vi "系统设置_古田户外.vi"() -> ()   [LabVIEW 2016]
uses:
  <vilib>/Utility/miscctls.llb/LVPointTypeDef.ctl
  <vilib>/Utility/config.llb/Read Key (U32).vi
  <vilib>/Utility/config.llb/Write Key (I32).vi
  PLC/PLC.lvlib
  <vilib>/ptbypt/NI_PtbyPt.lvlib
  <vilib>/Utility/config.llb/NI_LVConfig.lvlib
panel:
  in  "运行模式":enum16{"维护模式", "常规模式", "应急模式", "质控模式"}(ring)
  in  "运行间隔":i16=4 min=1 max=24
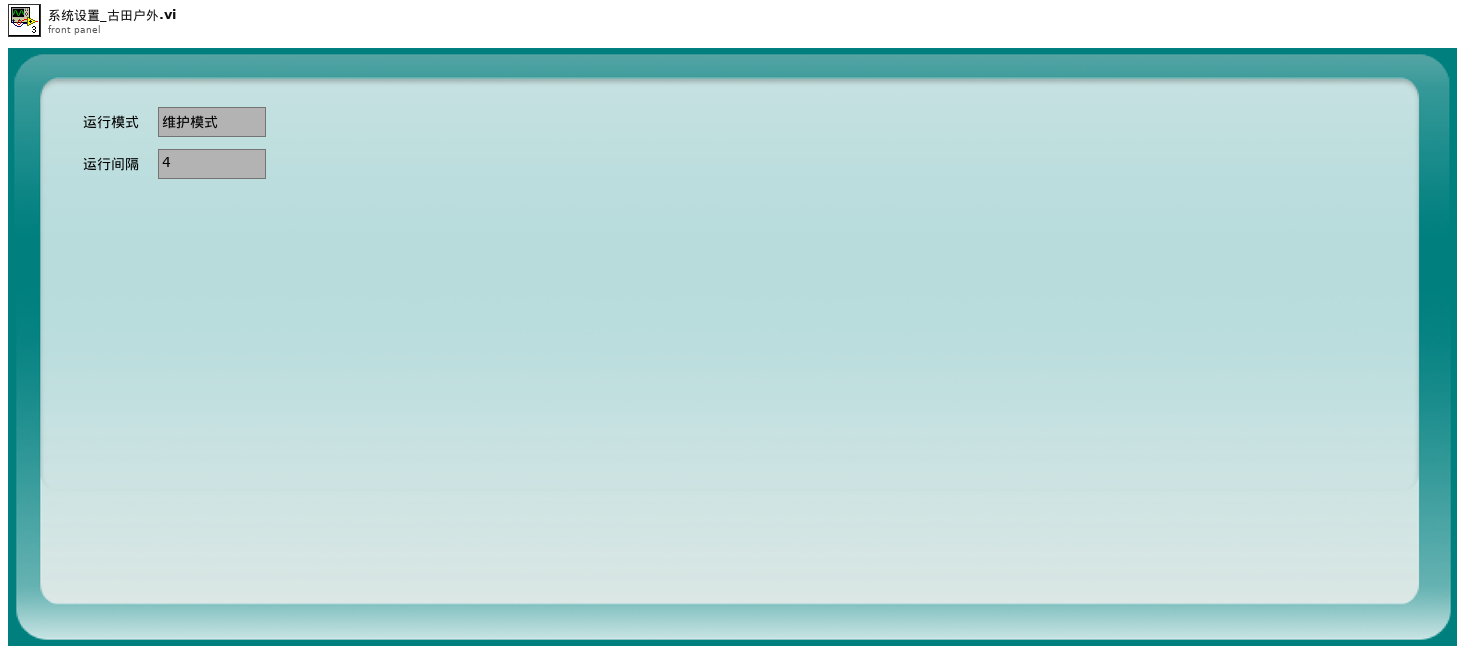
[diagram p1: front panel]
types:
  T1 = typedef "LVPointTypeDef.ctl" = cluster{"Horizontal":i16, "Vertical":i16}
  T2 = typedef "NI_LVConfig.lvlib/Config Data RefNum.ctl" = refnum<k1>
  T3 = enum16{"水样测量", "标样核查", "零点核查", "加标回收", "平行样", "校零", "校标"}
  T4 = cluster{"是否启用仪器":bool, "CODMn":cluster{"启动测量模式":cluster{"测量模式":enum16{"水样测量", "标样核查", "零点核查", "加标回收", "平行样", "校零", "校标"}}, "确定按钮":bool}}
  T5 = typedef "LVDateTimeRec.ctl" = cluster{"秒数的小数部分":dbl, "秒":i32, "分":i32, "时":i32, "日":i32, "月":i32, "年":i32, "天数（周）":i32, "天数（年）":i32, "DST":i32}
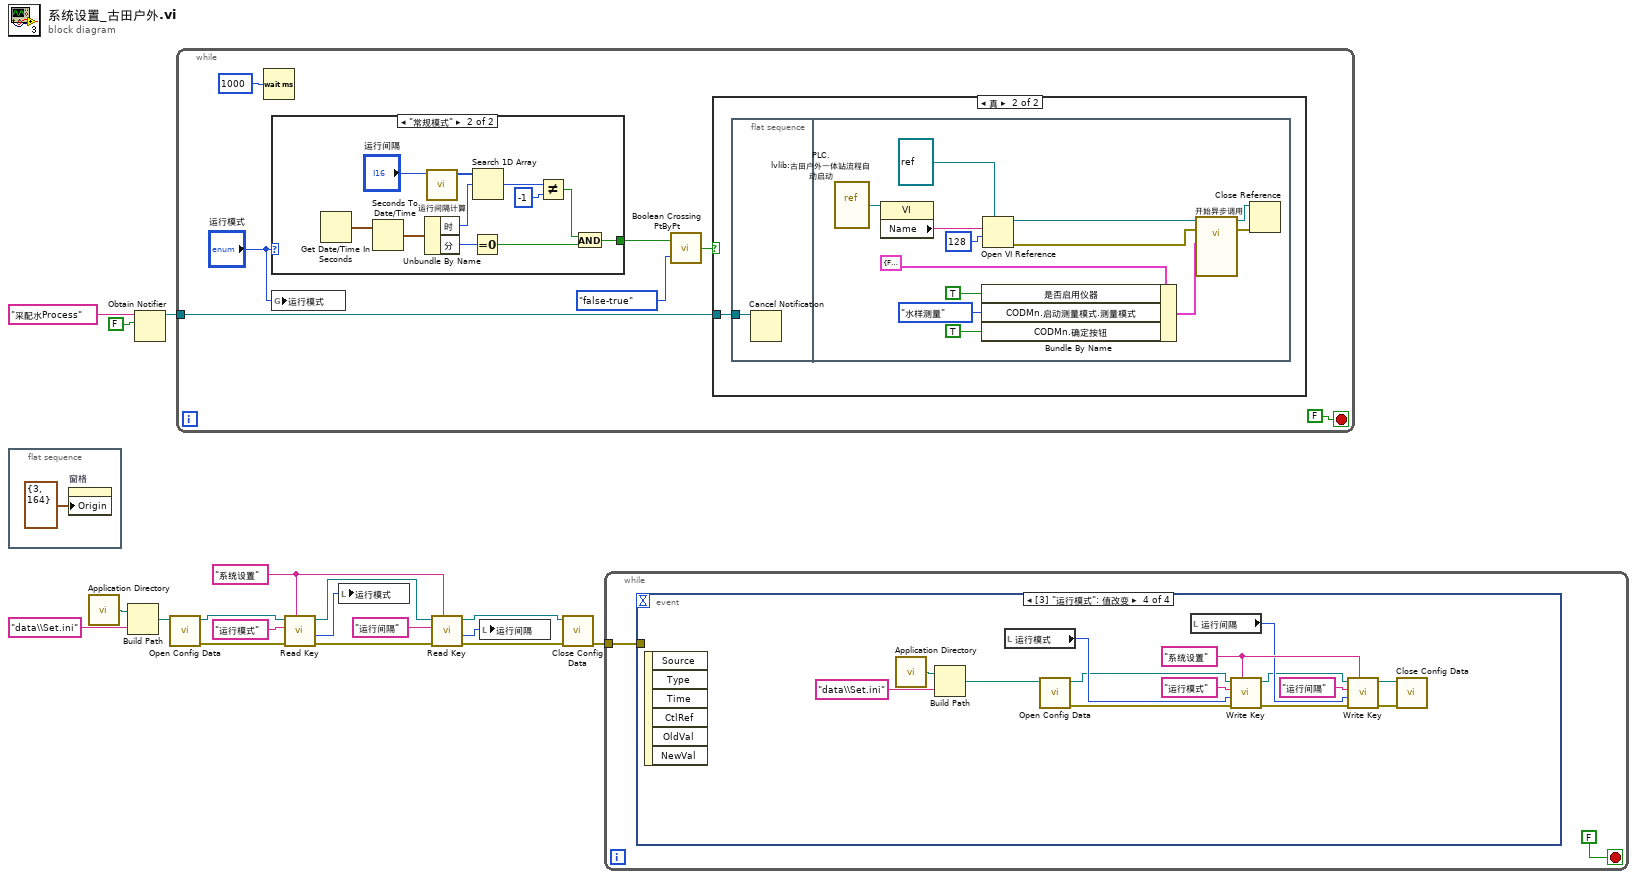
[diagram p0: block diagram]
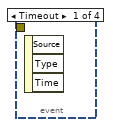
[diagram p4: hidden frame]
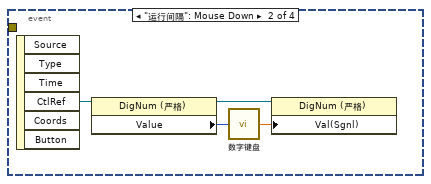
[diagram p5: hidden frame]
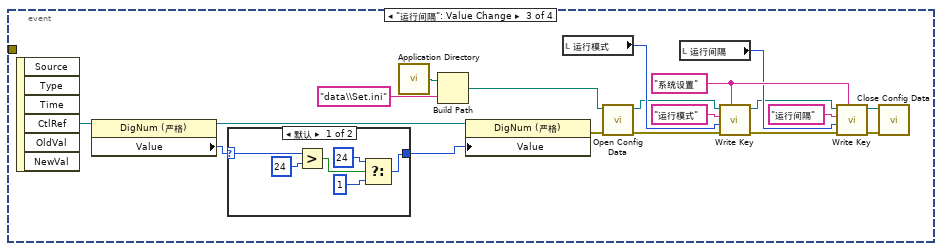
[diagram p6: hidden frame]
diagram:
  w1 = "系统设置" ("section")
  n1 = flat-sequence {
    frame #0 {
      n2 = property on="窗格" class="Pane"("Origin"=T1 {"Horizontal"=3, "Vertical"=164} ("原点")) -> ()  [unwired: 2 in, 2 out]
    }
  }
  n3 = call <vilib>:"Application Directory.vi"() -> ("Application Directory"=w13:path)
  n4 = Build Path(base path=w13, name or relative path="data\\Set.ini" ("名称或相对路径")) -> (appended path=w11:path)
  n5 = Obtain Notifier(name (unnamed)="采配水Process" ("名称（未命名）"), notification data type=FALSE) -> (notifier out=w16:refnum<notifier>)  [unwired: 2 in, 2 out]
  n6 = call <vilib>:"Open Config Data.vi"("configuration file path"=w11) -> ("error out"=w14:errorcluster, "refnum"=w15:T2)  [unwired: 8 in, 1 out]
  n7 = while {
    tunnel: w16 -> [w24]
    stop <- FALSE stop-if-true
    n8 = Wait (ms)(milliseconds to wait=u32 1000 ("等待时间（毫秒）")) -> ()  [unwired: 1 out]
    n9 = case shown="\"常规模式\"" "运行模式" {
      tunnel: [_ w42] -> w23
      frame "维护模式", Default {
      }
      frame "常规模式" {
        n10 = Get Date/Time In Seconds() -> (seconds since 1Jan1904=w51:timestamp)
        n11 = Seconds To Date/Time(time stamp (now)=w51) -> (date time rec=w50:T5)  [unwired: 1 in]
        n12 = Unbundle By Name(w50) -> ("时"=w47:i32, "分"=w49:i32)
        n13 = call "运行间隔计算.vi"("运行周期"="运行间隔") -> ("数组"=w48:i32[])  [unwired: 10 in]
        n14 = Equal To 0?(x=w49) -> (x = 0?=w43:bool)
        n15 = Search 1D Array(1D array=w48, element=w47) -> (index of element=w46:i32)  [unwired: 1 in]
        n16 = Not Equal?(x=w46, y=-1) -> (x != y?=w44:bool)
        n17 = And(x=w44, y=w43) -> (x .and. y?=w42:bool)
      }
    }
    n18 = global write "系统变量.vi" "运行模式"("运行模式") -> ()
    n19 = call <vilib>:"Boolean Crossing PtByPt.vi"("direction"=enum16{"either", "false-true", "true-false"}."false-true", "input"=w23) -> ("crossing"=w21:bool)  [unwired: 1 in]
    n20 = case shown="真" w21 {
      tunnel: w24 -> [_ w27]
      frame False {
      }
      frame True {
        n21 = flat-sequence {
          tunnel: w27 -> [w28]
          frame #0 {
            n22 = Cancel Notification(0:w28) -> ()  [unwired: 1 in, 3 out]
          }
          frame #1 {
            n23 = vi-ref "PLC.lvlib:古田户外一体站流程自动启动.vi"() -> (w41:refnum<vi>)
            n24 = property class="VI"(reference=w41) -> ("Name"=w40:string)  [unwired: 1 in, 2 out]
            n25 = Bundle By Name(cluster=T4 {"是否启用仪器"=FALSE, "CODMn"={"启动测量模式"={"测量模式"=enum."水样测量"}, "确定按钮"=FALSE}} ("参数"), "是否启用仪器"=TRUE, "CODMn.启动测量模式.测量模式"=T3."水样测量", "CODMn.确定按钮"=TRUE) -> (w30:T4)
            n26 = Open VI Reference(type specifier VI Refnum (for type only)=refnum<vi> refnum, vi path=w40, options=128 ("选项")) -> (vi reference=w38:refnum<vi>, error out=w35:errorcluster)  [unwired: 3 in]
            n27 = call-by-ref "开始异步调用"(reference=w38, error in=w35, "参数"=w30) -> (reference out=w36:refnum<vi>, error out=w34:errorcluster)  [unwired: 11 in]
            n28 = Close Reference(reference=w36, error in (no error)=w34) -> ()  [unwired: 1 out]
          }
        }
      }
    }
  }
  n29 = call-poly <vilib>:"Read Key.vi"("section"=w1, "error in (no error)"=w14, "key"="运行模式" ("section"), "refnum"=w15) -> ("error out"=w7:errorcluster, "value"=w10:u32, "refnum out"=w9:T2)  [unwired: 4 in, 1 out]
  n30 = local write "运行模式"(w10) -> ()
  n31 = call-poly <vilib>:"Read Key.vi"("section"=w1, "error in (no error)"=w7, "key"="运行间隔" ("section"), "refnum"=w9) -> ("error out"=w6:errorcluster, "value"=w3:u32, "refnum out"=w8:T2)  [unwired: 4 in, 1 out]
  n32 = local write "运行间隔"(w3) -> ()
  n33 = call <vilib>:"Close Config Data.vi"("error in (no error)"=w6, "refnum"=w8) -> ("error out"=w2:errorcluster)  [unwired: 8 in, 1 out]
  n34 = while {
    tunnel: w2 -> [w53]
    stop <- FALSE stop-if-true
    n35 = event shown="[3] \"运行模式\": 值改变" {
      selector: _ -> [_ _ _ _]
      dyn-events: _ -> [_ _ _ _]
      timeout: _ -> [_ _ _ _]
      tunnel: w53 -> [_ _ _ _]
      event Timeout {
        n36 = event-data() -> ()  [unwired: 1 in, 3 out]
      }
      event "运行间隔": Mouse Down {
        n37 = event-data() -> ("CtlRef"=w55:refnum<vi>)  [unwired: 1 in, 5 out]
        n38 = property class="DigNum (严格)"(reference=w55) -> (reference out=w57:refnum<vi>, "Value"=w56:i16)  [unwired: 1 in, 1 out]
        n39 = call "数字键盘.vi"("OldNumber"=w56) -> ("NewNumber"=w58:sgl)
        n40 = property class="DigNum (严格)"(reference=w57, "Val(Sgnl)"=w58) -> ()  [unwired: 1 in, 2 out]
      }
      event "运行间隔": Value Change {
        w73 = "系统设置" ("section")
        n41 = event-data() -> ("CtlRef"=w77:refnum<vi>)  [unwired: 1 in, 5 out]
        n42 = property class="DigNum (严格)"(reference=w77) -> (reference out=w75:refnum<vi>, "Value"=w76:i16)  [unwired: 1 in, 1 out]
        n43 = case shown="默认" w76 {
          selector: w76 -> [w80 w84]
          tunnel: [w79 w84] -> w74
          frame Default {
            n44 = Greater?(x=w80, y=i16 24) -> (0:w82:bool)
            n45 = Select(t=i16 24 ("y"), s=w82, f=i16 1) -> (s? t:f=w79:i16)
          }
          frame 1..24 {
          }
        }
        n46 = call <vilib>:"Application Directory.vi"() -> ("Application Directory"=w68:path)
        n47 = Build Path(base path=w68, name or relative path="data\\Set.ini" ("名称或相对路径")) -> (appended path=w66:path)
        n48 = property class="DigNum (严格)"(reference=w75, "Value"=w74) -> (error out=w59:errorcluster)  [unwired: 1 in, 1 out]
        n49 = local read "运行模式"() -> (w71:enum16{"维护模式", "常规模式", "应急模式", "质控模式"})
        n50 = call <vilib>:"Open Config Data.vi"("error in (no error)"=w59, "configuration file path"=w66) -> ("error out"=w69:errorcluster, "refnum"=w70:T2)  [unwired: 7 in, 1 out]
        n51 = local read "运行间隔"() -> (w72:i16)
        n52 = call-poly <vilib>:"Write Key.vi"("section"=w73, "error in (no error)"=w69, "value"=w71, "key"="运行模式" ("section"), "refnum"=w70) -> ("error out"=w63:errorcluster, "refnum out"=w65:T2)  [unwired: 4 in, 1 out]
        n53 = call-poly <vilib>:"Write Key.vi"("section"=w73, "error in (no error)"=w63, "value"=w72, "key"="运行间隔" ("section"), "refnum"=w65) -> ("error out"=w62:errorcluster, "refnum out"=w64:T2)  [unwired: 4 in, 1 out]
        n54 = call <vilib>:"Close Config Data.vi"("error in (no error)"=w62, "refnum"=w64) -> ()  [unwired: 8 in, 2 out]
      }
      event "运行模式": Value Change {
        w98 = "系统设置" ("section")
        n55 = event-data() -> ()  [unwired: 1 in, 6 out]
        n56 = call <vilib>:"Application Directory.vi"() -> ("Application Directory"=w93:path)
        n57 = Build Path(base path=w93, name or relative path="data\\Set.ini" ("名称或相对路径")) -> (appended path=w91:path)
        n58 = local read "运行模式"() -> (w96:enum16{"维护模式", "常规模式", "应急模式", "质控模式"})
        n59 = call <vilib>:"Open Config Data.vi"("configuration file path"=w91) -> ("error out"=w94:errorcluster, "refnum"=w95:T2)  [unwired: 8 in, 1 out]
        n60 = local read "运行间隔"() -> (w97:i16)
        n61 = call-poly <vilib>:"Write Key.vi"("section"=w98, "error in (no error)"=w94, "value"=w96, "key"="运行模式" ("section"), "refnum"=w95) -> ("error out"=w88:errorcluster, "refnum out"=w90:T2)  [unwired: 4 in, 1 out]
        n62 = call-poly <vilib>:"Write Key.vi"("section"=w98, "error in (no error)"=w88, "value"=w97, "key"="运行间隔" ("section"), "refnum"=w90) -> ("error out"=w87:errorcluster, "refnum out"=w89:T2)  [unwired: 4 in, 1 out]
        n63 = call <vilib>:"Close Config Data.vi"("error in (no error)"=w87, "refnum"=w89) -> ()  [unwired: 8 in, 2 out]
      }
    }
  }
